vi "GPS Wait for Valid Data.vi"(3 "error in (no error)":errorcluster, 5 "Completed NMEA Sentences":string[](array[string])) -> (0 "error out":errorcluster, 1 "Valid Data":bool, 2 "Complete NMEA Sentences (Copy)":string[](array[string]))   [LabVIEW 2009]
uses:
  <vilib>/robotics/Protocols/NMEA/Advanced/Instrument Specific Poly VIs/GPS/Parse GGA Sentence.vi
  <vilib>/robotics/Protocols/NMEA/NMEA API.lvlib
panel:
  out "Heartbeat":bool
  out "input array size":i32
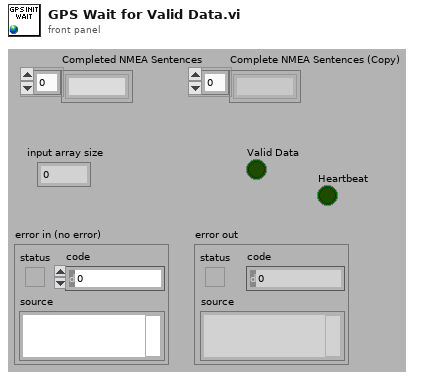
[diagram p1: front panel]
types:
  T1 = typedef "NMEA API.lvlib/GGA Data.ctl" = cluster{"time of fix":cluster{"included?":bool, "time (UTC)":timestamp}, "latitude":cluster{"included?":bool, "latitude (deg)":dbl}, "longitude":cluster{"included?":bool, "longitude (deg)":dbl}, "fix quality":cluster{"included?":bool, "quality":u16}, "number of satellites in view":cluster{"included?":bool, "number of satellites":i8}, "horizontal dilution of precision":cluster{"included?":bool, "horizontal DOP":dbl}, "altitude above mean sea level":cluster{"included?":bool, "altitude (m)":dbl}, "height of geoid above WGS84":cluster{"included?":bool, "height of geoid (m)":dbl}, "time since last DGPS update":cluster{"included?":bool, "time (s)":dbl}, "DGPS station ID number":cluster{"included?":bool, "station ID number":dbl}}
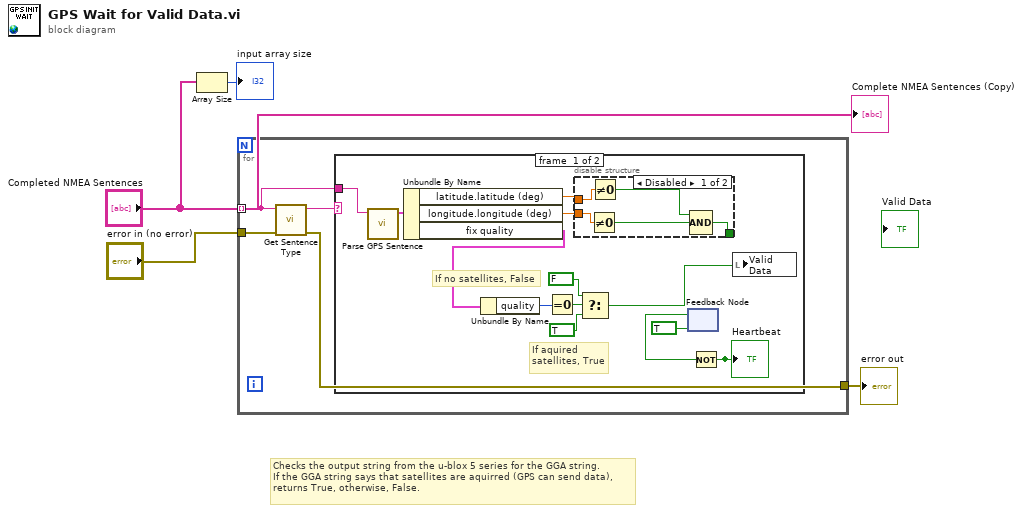
[diagram p0: block diagram]
diagram:
  # "Checks the output string from the u-blox 5 series for the GGA string.\nIf the GGA string says that satellites are aquirred (GPS can send data),\nreturns True, otherwise, False."
  n1 = Array Size(array="Completed NMEA Sentences") -> (size(s)=→"input array size":i32)
  n2 = for {
    tunnel: "Completed NMEA Sentences" -> [w6] mode=indexing
    tunnel: "error in (no error)" -> [w8]
    tunnel: [w5] -> w1
    n3 = call <vilib>:"Get Sentence Type.vi"("error in (no error)"=w8, "sentence"=w6) -> ("error out"=w5:errorcluster, "sentence type"=w7:string)  [unwired: 7 in, 1 out]
    n4 = case shown="\"GPGGA\"" w7 {
      tunnel: w6 -> [w21 _]
      frame #0 {
        # "If no satellites, False"
        # "If aquired \nsatellites, True"
        n5 = call-poly <vilib>:"Parse GPS Sentence.vi"("GGA sentence"=w21) -> ("GGA data"=w16:T1)  [unwired: 9 in, 1 out]
        n6 = Unbundle By Name(w16) -> ("latitude.latitude (deg)"=w13:dbl, "longitude.longitude (deg)"=w14:dbl, "fix quality"=w15:cluster{"included?":bool, "quality":u16})
        n7 = Unbundle By Name(w15) -> ("quality"=w17:u16)
        n8 = Equal To 0?(x=w17) -> (x = 0?=w20:bool)
        n9 = disable-structure shown="Disabled" {
          disable-tunnel: w14 -> [w26 _]
          disable-tunnel: w13 -> [w23 _]
          disable-tunnel: [w22 _] -> _
          frame #0 {
            n10 = Not Equal To 0?(x=w26) -> (x != 0?=w25:bool)
            n11 = Not Equal To 0?(x=w23) -> (x != 0?=w24:bool)
            n12 = Compound Arithmetic op=AND(w24, w25) -> (w22:bool)  [unwired: 1 in]
          }
          frame #1 {
          }
        }
        n13 = Select(t=FALSE, s=w20, f=TRUE) -> (s? t:f=w12:bool)
        n14 = feedback #1(TRUE) -> (w10:bool)
        n15 = Not(x=w10) -> (.not. x?=w9:bool)
        "Heartbeat" <- w9
        n16 = local write "Valid Data"(w12) -> ()
      }
      frame #1 {
      }
    }
  }
  "error out" <- w1
  "Complete NMEA Sentences (Copy)" <- "Completed NMEA Sentences"
